vi "gRPC Client Test.vi"() -> ()   [LabVIEW 2021, in "basic_switch_executive_driver_client.lvlib"]
uses:
  basic_switch_executive_driver_client.lvlib
  RPC Messages/nise_OpenSessionInputs.ctl
  <vilib>/Plug-In SDKs/Clients/Session Management V1/Session Reservation/Initialize and Close Session Behavior.ctl
  RPC Messages/nise_StatusInfo.ctl
  <vilib>/gRPC/Generated APIs/ni/measurementlink/discovery/v1/RPC Messages/ni_measurementlink_discovery_v1_ResolveServiceRequest.ctl
  RPC Messages/nise_ConnectInfo.ctl
  RPC Messages/nise_SessionInformation.ctl
  RPC Messages/nise_MulticonnectMode.ctl
  RPC Messages/nise_DisconnectInfo.ctl
  <vilib>/Plug-In SDKs/Clients/Discovery V1/NI Discovery V1 Client.lvlib
  <vilib>/gRPC/Generated APIs/ni/measurementlink/discovery/v1/ni.measurementlink.discovery.v1.api.lvlib
  <vilib>/Plug-In SDKs/Clients/Session Management V1/Session Reservation/Session Reservation.lvclass
panel:
  out "error out":errorcluster
  out "Response Data":T1
  in  "Open Request Data":T2={"virtual_device_name"="VirtualDevice1", "optional_string"="", "initialize_and_close_session_behavior"=enum."Initialize and Detach"}
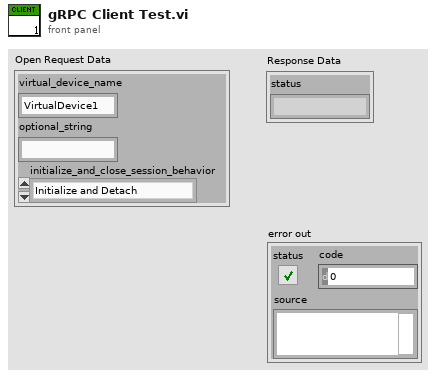
[diagram p1: front panel]
types:
  T1 = typedef "basic_switch_executive_driver_client.lvlib/nise_StatusInfo.ctl" = cluster{"status":string}
  T2 = typedef "basic_switch_executive_driver_client.lvlib/nise_OpenSessionInputs.ctl" = cluster{"virtual_device_name":string, "optional_string":string, "initialize_and_close_session_behavior":T3}
  T3 = typedef "NI Session Management V1 Client.lvlib/Session Reservation.lvclass/Initialize and Close Session Behavior.ctl" = enum16{"Auto", "Initialize and Close", "Attach and Detach", "Initialize and Detach", "Attach and Close"}
  T4 = typedef "basic_switch_executive_driver_client.lvlib/nise_ConnectInfo.ctl" = cluster{"connection_specification":string, "session_info":T5, "wait_for_rebounce":bool, "multi_connect_mode":T6}
  T5 = typedef "basic_switch_executive_driver_client.lvlib/nise_SessionInformation.ctl" = cluster{"session_id":u32, "initialize_and_close_session_behavior":T3}
  T6 = typedef "basic_switch_executive_driver_client.lvlib/nise_MulticonnectMode.ctl" = enum32{"NO_MULTICONNECT", "USE_DEFAULT_MODE", "MULTICONNECT_ROUTES"}
  T7 = typedef "ni.measurementlink.discovery.v1.api.lvlib/ni_measurementlink_discovery_v1_ResolveServiceRequest.ctl" = cluster{"provided_interface":string, "service_class":string, "deployment_target":string, "version":string}
  T8 = typedef "basic_switch_executive_driver_client.lvlib/nise_DisconnectInfo.ctl" = cluster{"disconnect_specification":string, "session_info":T5}
  T9 = typedef "ni.measurementlink.discovery.v1.api.lvlib/ni_measurementlink_discovery_v1_ServiceLocation.ctl" = cluster{"location":string, "insecure_port":string, "ssl_authenticated_port":string}
  T10 = typedef "grpc-lvsupport-release.lvlib/grpcId.ctl" = u64
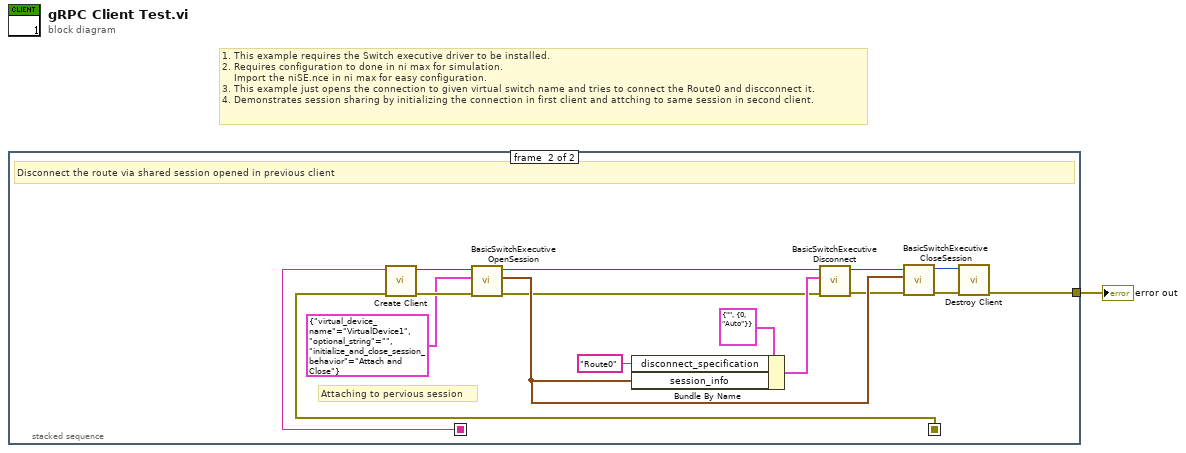
[diagram p0: block diagram]
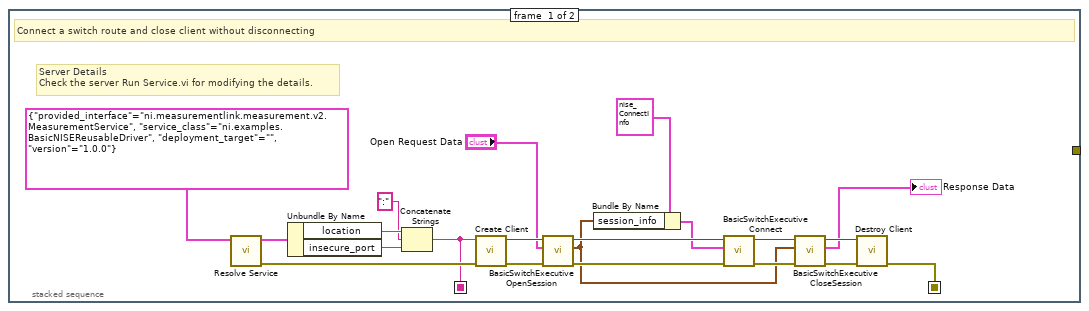
[diagram p2: hidden frame]
diagram:
  # "1. This example requires the Switch executive driver to be installed.\n2. Requires configuration to done in ni max for simulation.\n    Import the niSE.nce in ni max for easy configuration. \n3. This example just opens the connection to given virtual switch name and tries to connect the Route0 and discconnect it.\n4. Demonstrates session sharing by initializing the connection in first client and attching to same session in second client."
  n1 = stacked-sequence {
    seq-local: [w3 _] -> [_ w25]
    seq-local: [w2 _] -> [_ w24]
    tunnel: [_ w23] -> w1
    frame #0 {
      # "Server Details\nCheck the server Run Service.vi for modifying the details."
      # "Connect a switch route and close client without disconnecting"
      n2 = call <vilib>:"Resolve Service.vi"("request data"=T7 {"provided_interface"="ni.measurementlink.measurement.v2.MeasurementService", "service_class"="ni.examples.BasicNISEReusableDriver", "deployment_target"="", "version"="1.0.0"}) -> ("error out"=w4:errorcluster, "response data"=w8:T9)  [unwired: 9 in]
      n3 = Unbundle By Name(w8) -> ("location"=w6:string, "insecure_port"=w7:string)
      n4 = Concatenate Strings(w6, ":" ("string"), w7) -> (w2:string)
      n5 = call "Create Client.vi"("error in"=w4, "address"=w2) -> ("error out"=w21:errorcluster, "gRPC ID Out"=w22:T10)  [unwired: 8 in]
      n6 = call "BasicSwitchExecutive OpenSession.vi"("error in"=w21, "Request Data"="Open Request Data", "gRPC ID"=w22) -> ("error out"=w15:errorcluster, "Response Data"=w11:T5, "gRPC ID out"=w16:T10)  [unwired: 6 in]
      n7 = Bundle By Name(cluster=T4 {"connection_specification"="Route0", "session_info"={"session_id"=0, "initialize_and_close_session_behavior"=enum."Auto"}, "wait_for_rebounce"=FALSE, "multi_connect_mode"=enum."USE_DEFAULT_MODE"} ("Conn Request Data"), "session_info"=w11) -> (w12:T4)
      n8 = call "BasicSwitchExecutive Connect.vi"("error in"=w15, "Request Data"=w12, "gRPC ID"=w16) -> ("error out"=w13:errorcluster, "gRPC ID out"=w14:T10)  [unwired: 6 in, 1 out]
      n9 = call "BasicSwitchExecutive CloseSession.vi"("error in"=w13, "Request Data"=w11, "gRPC ID"=w14) -> ("error out"=w20:errorcluster, "Response Data"=→"Response Data":T1, "gRPC ID out"=w19:T10)  [unwired: 6 in]
      n10 = call "Destroy Client.vi"("error in"=w20, "gRPC ID"=w19) -> ("error out"=w3:errorcluster)  [unwired: 9 in]
    }
    frame #1 {
      # "Attaching to pervious session"
      # "Disconnect the route via shared session opened in previous client"
      n11 = call "Create Client.vi"("error in"=w25, "address"=w24) -> ("error out"=w29:errorcluster, "gRPC ID Out"=w30:T10)  [unwired: 8 in]
      n12 = call "BasicSwitchExecutive OpenSession.vi"("error in"=w29, "Request Data"=T2 {"virtual_device_name"="VirtualDevice1", "optional_string"="", "initialize_and_close_session_behavior"=enum."Attach and Close"}, "gRPC ID"=w30) -> ("error out"=w31:errorcluster, "Response Data"=w36:T5, "gRPC ID out"=w32:T10)  [unwired: 6 in]
      n13 = Bundle By Name(cluster=T8 {"disconnect_specification"="", "session_info"={"session_id"=0, "initialize_and_close_session_behavior"=enum."Auto"}} ("Request Data"), "disconnect_specification"="Route0", "session_info"=w36) -> (w33:T8)
      n14 = call "BasicSwitchExecutive Disconnect.vi"("error in"=w31, "Request Data"=w33, "gRPC ID"=w32) -> ("error out"=w35:errorcluster, "gRPC ID out"=w34:T10)  [unwired: 6 in, 1 out]
      n15 = call "BasicSwitchExecutive CloseSession.vi"("error in"=w35, "Request Data"=w36, "gRPC ID"=w34) -> ("error out"=w37:errorcluster, "gRPC ID out"=w38:T10)  [unwired: 6 in, 1 out]
      n16 = call "Destroy Client.vi"("error in"=w37, "gRPC ID"=w38) -> ("error out"=w23:errorcluster)  [unwired: 9 in]
    }
  }
  "error out" <- w1
